vi "Write System Timing Model.vi"(8 "error in (no error)":errorcluster, 10 "system timing model":T1=10178 items=["Finite"=10178, "-"=-1, "Continuous"=10123, "-"=-2, "Settled"=110123, "Averaged"=210123, "Discrete Sweep"=310123, "Continuous Sweep"=410123], 11 "signal configuration":refnum<class "SV Signal.lvclass">) -> (0 "error out":errorcluster, 3 "signal configuration":refnum<class "SV Signal.lvclass">)   [LabVIEW 2017, in "SV Signal.lvclass"]
uses:
  <vilib>/addons/_NISVFA/_Generation/Signal Generation/SV Signal/SV Signal.lvclass
  <vilib>/addons/_NISVFA/_Generation/Signal Generation/SV Signal/sv_System Timing Model.ctl
  <vilib>/addons/_NISVFA/_Generation/Signal Generation/SV Signal/SV Signal.lvclass/SV Signal.ctl
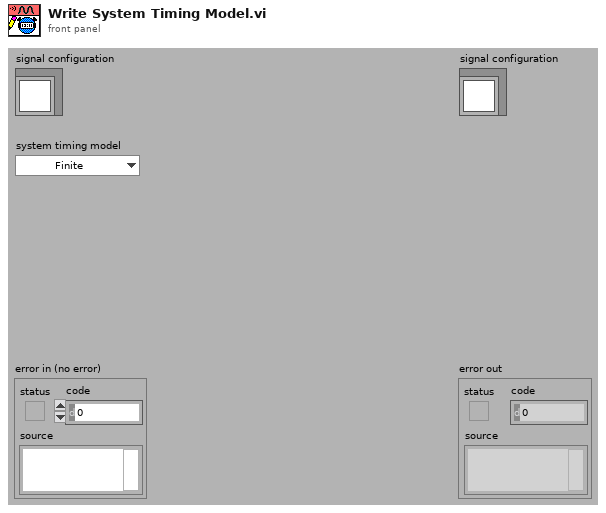
[diagram p1: front panel]
types:
  T1 = typedef "SV Signal.lvclass/sv_System Timing Model.ctl" = i64
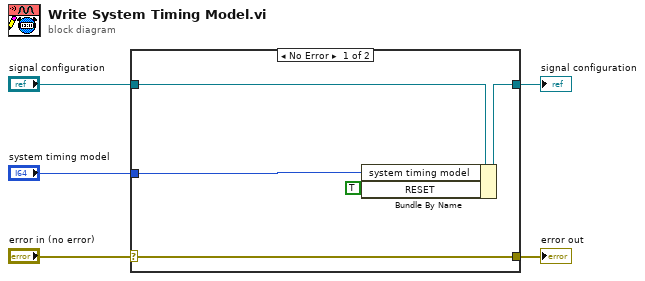
[diagram p0: block diagram]
diagram:
  n1 = case shown="No Error" "error in (no error)" {
    selector: "error in (no error)" -> [w10 w11]
    tunnel: [w10 w11] -> w4
    tunnel: [w8 w12] -> w2
    tunnel: "signal configuration" -> [w9 w12]
    tunnel: "system timing model" -> [w7 _]
    frame No Error {
      n2 = Bundle By Name(cluster=w9, "system timing model"=w7, "RESET"=TRUE ("state.RESET")) -> (w8:refnum<class "SV Signal.lvclass">)
    }
    frame Error {
    }
  }
  "error out" <- w4
  "signal configuration" <- w2
